vi "VisionNetworkSlowRead.vi"(8 "error in (no error)":errorcluster) -> (0 "error out":errorcluster)   [LabVIEW 2023]
doc: "Vision Network\n\nInput\n --Error in \n\nOutput\n --Error out"
uses:
  <vilib>/Rock Robotics/WPI/ThirdParty/JAS_Junk/TrajLib/Rotation2d_CreateAngle.vi
  <vilib>/Rock Robotics/WPI/ThirdParty/JAS_Junk/TrajLib/Translation2d_Create.vi
  <vilib>/Rock Robotics/Network Tables/NT Read Number.vi
  VisionGlobal.vi
  <vilib>/Rock Robotics/WPI/ThirdParty/JAS_Junk/TrajLib/Trajectory_Library.lvlib
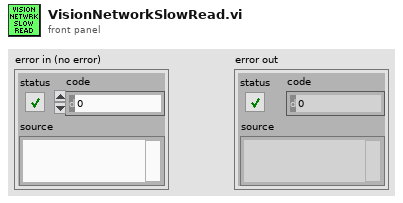
[diagram p1: front panel]
types:
  T1 = typedef "Trajectory_Library.lvlib/POSE2D.ctl" = cluster{"TRANSLATION":T2, "ROTATION":T3}
  T2 = typedef "Trajectory_Library.lvlib/TRANSLATION2D.ctl" = cluster{"X":dbl, "Y":dbl}
  T3 = typedef "Trajectory_Library.lvlib/ROTATION2D.ctl" = cluster{"VALUE":dbl, "COS":dbl, "SIN":dbl}
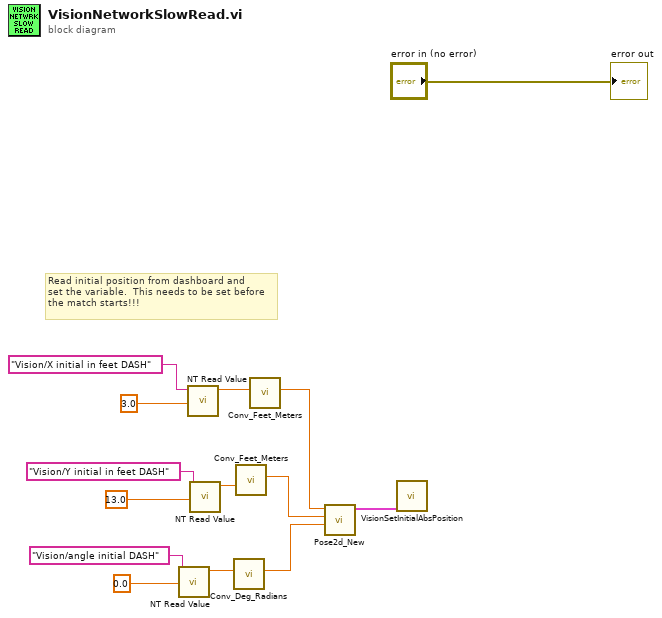
[diagram p0: block diagram]
diagram:
  # "Read initial position from dashboard and\nset the variable.  This needs to be set before\nthe match starts!!!"
  n1 = call-poly <vilib>:"NT Read Value.vi"("default value"=0.0, "name"="Vision/angle initial DASH") -> ("value"=w8:dbl)  [unwired: 7 in, 2 out]
  n2 = call-poly <vilib>:"NT Read Value.vi"("default value"=3.0, "name"="Vision/X initial in feet DASH") -> ("value"=w11:dbl)  [unwired: 7 in, 2 out]
  n3 = call-poly <vilib>:"NT Read Value.vi"("default value"=13.0, "name"="Vision/Y initial in feet DASH") -> ("value"=w10:dbl)  [unwired: 7 in, 2 out]
  n4 = call <vilib>:"Conv_Deg_Radians.vi"("Degress"=w8) -> ("Radians"=w7:dbl)  [unwired: 10 in]
  n5 = call <vilib>:"Conv_Feet_Meters.vi"("Feet"=w10) -> ("Meters"=w9:dbl)  [unwired: 10 in]
  n6 = call <vilib>:"Conv_Feet_Meters.vi"("Feet"=w11) -> ("Meters"=w12:dbl)  [unwired: 10 in]
  n7 = call <vilib>:"Pose2d_New.vi"("Heading"=w7, "Y"=w9, "X"=w12) -> ("out POSe"=w13:T1)  [unwired: 8 in]
  n8 = call "VisionSetInitialAbsPosition.vi"("InitialPose"=w13) -> ()  [unwired: 11 in]
  "error out" <- "error in (no error)"
